vi "Extract Packet Identifier.vi"(11 "Control Packet":u8[](array[numeric]) format="%08b") -> (2 "Valid":bool, 3 "Control Packet Type":T1)   [LabVIEW 2013]
uses:
  Control Packet Type -- enum.ctl
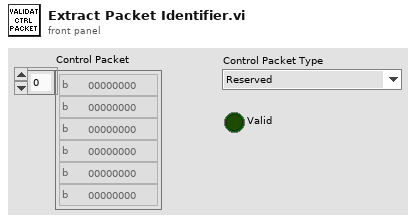
[diagram p1: front panel]
types:
  T1 = typedef "Control Packet Type -- enum.ctl" = enum16{"Reserved", "CONNECT", "CONNACK", "PUBLISH", "PUBACK", "PUBREC", "PUBREL", "PUBCOMP", "SUBSCRIBE", "SUBACK", "UNSUBSCRIBE", "UNSUBACK", "PINGREQ", "PINGRESP", "DISCONNECT", "Reserved(15)"}
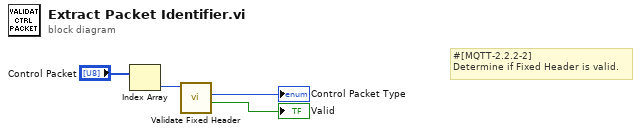
[diagram p0: block diagram]
diagram:
  # "#[MQTT-2.2.2-2]\nDetermine if Fixed Header is valid."
  n1 = Index Array(array="Control Packet") -> (element=w3:u8)  [unwired: 1 in]
  n2 = call "Validate Fixed Header.vi"("Fixed Header"=w3) -> ("Valid"=→"Valid":bool, "Control Packet Type"=→"Control Packet Type":T1)  [unwired: 8 in, 1 out]
